vi "AODO-Initialize DO.vi"(0 "DO":T2, 7 "Sync Task":refnum<k21>, 9 "initialized array":bool[][](array[boolean]), 11 "error in (no error)":errorcluster) -> (4 "DO Tasks":T1, 15 "error out":errorcluster)   [LabVIEW 2020]
uses:
  Typedefs/DO-Output Spec.ctl
  Typedefs/AODO-DO Tasks.ctl
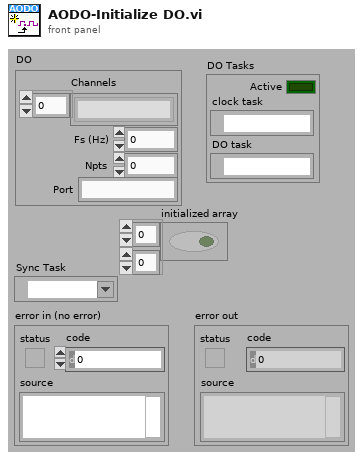
[diagram p1: front panel]
types:
  T1 = typedef "AODO-DO Tasks.ctl" = cluster{"Active":bool, "clock task":refnum<k21>, "DO task":refnum<k21>}
  T2 = typedef "DO-Output Spec.ctl" = cluster{"Channels":string[], "Fs (Hz)":dbl, "Npts":i32, "Port":string}
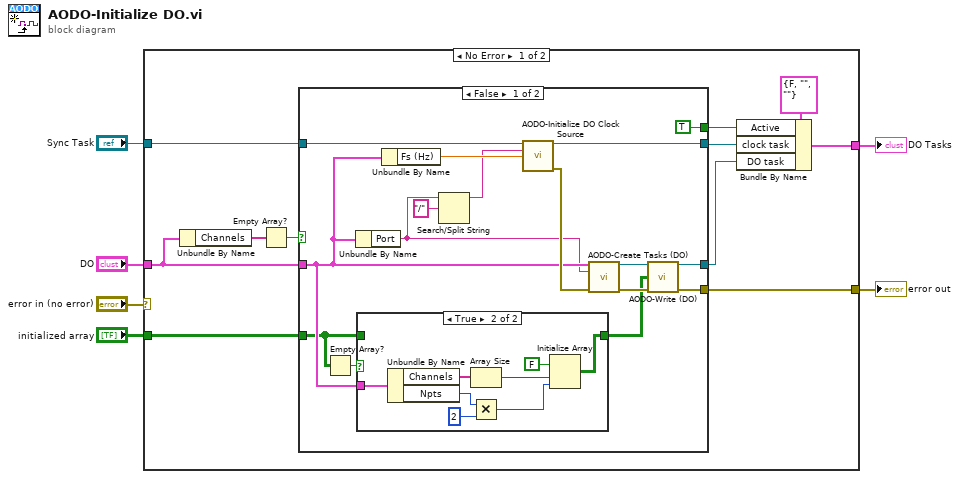
[diagram p0: block diagram]
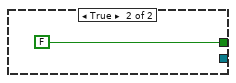
[diagram p3: hidden frame]
diagram:
  n1 = case shown="No Error" "error in (no error)" {
    selector: "error in (no error)" -> [_ w44]
    tunnel: [w17 w44] -> w6
    tunnel: "DO" -> [w15 _]
    tunnel: "Sync Task" -> [w16 _]
    tunnel: [w9 _] -> w2
    tunnel: "initialized array" -> [w7 _]
    frame No Error {
      n2 = Unbundle By Name(w15) -> ("Channels"=w14:string[])
      n3 = Empty Array?(array=w14) -> (empty?=w13:bool)
      n4 = case shown="False" w13 {
        tunnel: [w25 _] -> w17
        tunnel: w16 -> [w33 _]
        tunnel: w15 -> [w24 _]
        tunnel: [w30 _] -> w12
        tunnel: [w26 _] -> w11
        tunnel: [TRUE FALSE] -> w10
        tunnel: w7 -> [w20 _]
        frame False {
          n5 = Empty Array?(array=w20) -> (empty?=w19:bool)
          n6 = Unbundle By Name(w24) -> ("Port"=w21:string)
          n7 = case shown="True" w19 {
            tunnel: w24 -> [_ w36]
            tunnel: w20 -> [w34 _]
            tunnel: [w34 w35] -> w18
            frame False {
            }
            frame True {
              n8 = Unbundle By Name(w36) -> ("Channels"=w40:string[], "Npts"=w39:i32)
              n9 = Array Size(array=w40) -> (size(s)=w41:i32)
              n10 = Multiply(x=w39, y=2) -> (x*y=w37:i32)
              n11 = Initialize Array(FALSE, w41, w37) -> (w35:bool[][])
            }
          }
          n12 = Unbundle By Name(w24) -> ("Fs (Hz)"=w32:dbl)
          n13 = Search/Split String(string=w21, search string/char (-)="/") -> (substring before match=w22:string)  [unwired: 1 in, 2 out]
          n14 = call "AODO-Initialize DO Clock Source.vi"("Sync Task"=w33, "DAQmx Device Name"=w22, "Fs (Hz)"=w32) -> ("clock task"=w30:refnum<k21>, "error out"=w31:errorcluster)  [unwired: 11 in]
          n15 = call "AODO-Create Tasks (DO).vi"("DO"=w24, "DAQmx Device Name"=w21, "error in"=w31) -> ("task out"=w27:refnum<k21>, "error out"=w28:errorcluster)  [unwired: 11 in]
          n16 = call "AODO-Write (DO).vi"("Task In"=w27, "DO Waveforms"=w18, "error in (no error)"=w28) -> ("Task Out"=w26:refnum<k21>, "error out"=w25:errorcluster)  [unwired: 11 in]
        }
        frame True {
        }
      }
      n17 = Bundle By Name(cluster=T1 {"Active"=FALSE, "clock task"="", "DO task"=""} ("DO Tasks"), "Active"=w10, "clock task"=w12, "DO task"=w11) -> (w9:T1)
    }
    frame Error {
    }
  }
  "error out" <- w6
  "DO Tasks" <- w2
